vi "FindProjectElement.vi"(10 "Element name":string, 11 "Project item":refnum<vi>) -> (0 "Error":errorcluster, 2 "Found":bool, 3 "Element out":refnum<vi>)   [LabVIEW 2021, in "Tree.lvlib" / "Tree.lvclass"]
uses:
  Tree.lvclass
  Tree.lvclass/Tree.ctl
panel:
  # "Ищет в проекте объект (vi, класс, папка и т.д.) с названием Element name"
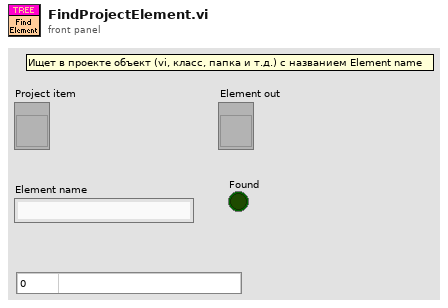
[diagram p1: front panel]
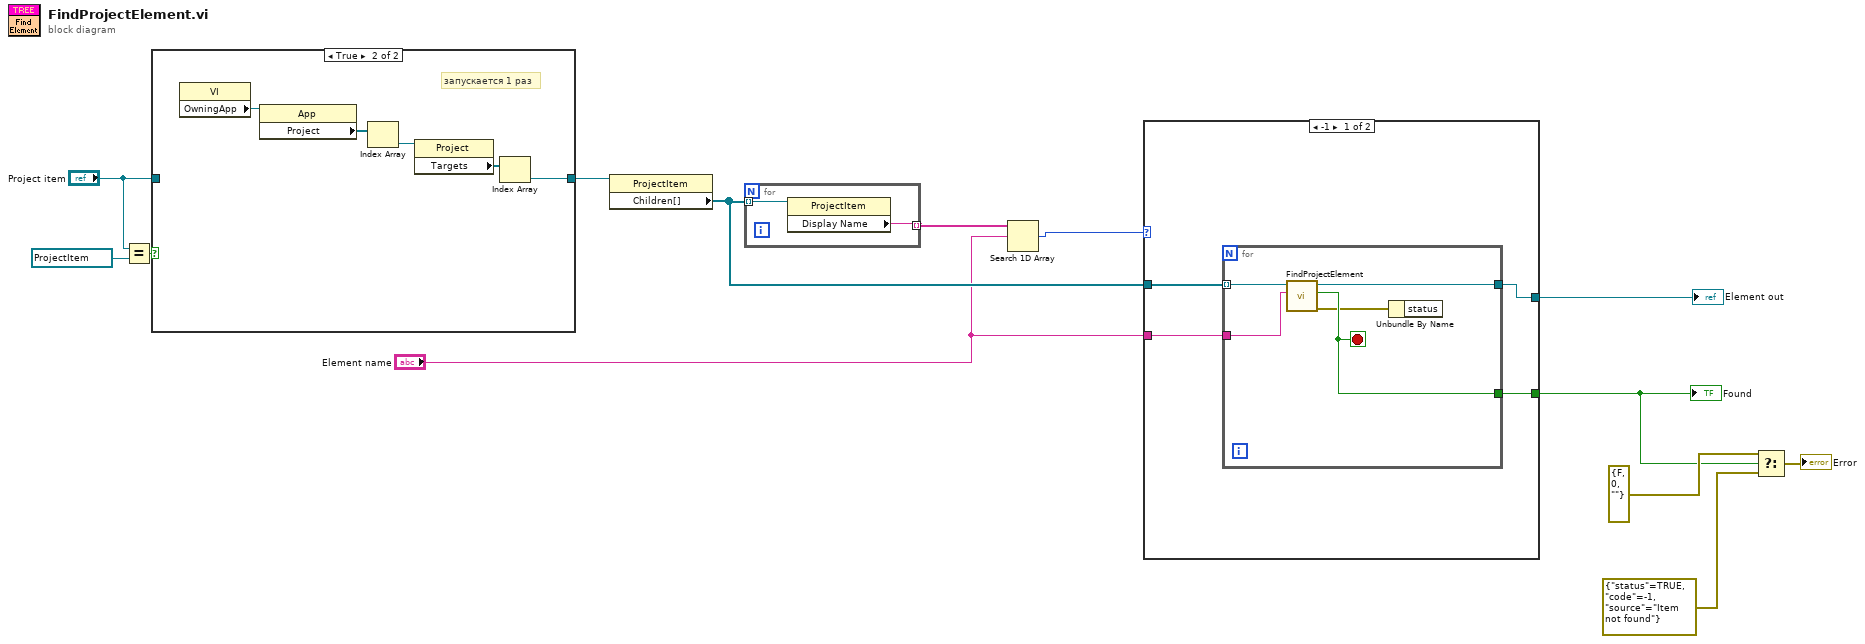
[diagram p0: block diagram]
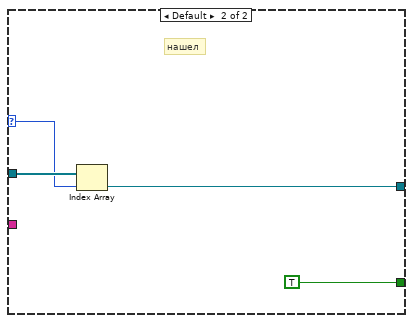
[diagram p3: hidden frame]
diagram:
  n1 = Equal?(x="Project item", y=refnum<vi> refnum) -> (x = y?=w3:bool)
  n2 = case shown="True" w3 {
    tunnel: [w14 w15] -> w2
    tunnel: "Project item" -> [w14 _]
    frame False {
    }
    frame True {
      # "запускается 1 раз"
      n3 = property class="VI"() -> ("OwningApp"=w16:refnum<vi>)  [unwired: 2 in, 2 out]
      n4 = property class="App"(reference=w16) -> ("Project"=w17:refnum<vi>[])  [unwired: 1 in, 2 out]
      n5 = Index Array(array=w17) -> (element=w18:refnum<vi>)  [unwired: 1 in]
      n6 = property class="Project"(reference=w18) -> ("Targets"=w19:refnum<vi>[])  [unwired: 1 in, 2 out]
      n7 = Index Array(array=w19) -> (element=w15:refnum<vi>)  [unwired: 1 in]
    }
  }
  n8 = property class="ProjectItem"(reference=w2) -> ("Children[]"=w11:refnum<vi>[])  [unwired: 1 in, 2 out]
  n9 = for {
    tunnel: w11 -> [w20] mode=indexing
    tunnel: [w21] -> w13 mode=indexing
    n10 = property class="ProjectItem"(reference=w20) -> ("Display Name"=w21:string)  [unwired: 1 in, 2 out]
  }
  n11 = Search 1D Array(1D array=w13, element="Element name") -> (index of element=w9:i32)  [unwired: 1 in]
  n12 = case shown="-1" w9 {
    selector: w9 -> [_ w31]
    tunnel: [w23 w34] -> w12
    tunnel: w11 -> [w25 w33]
    tunnel: "Element name" -> [w24 _]
    tunnel: [w22 TRUE ("Found")] -> w5
    frame -1 {
      n13 = for {
        tunnel: w25 -> [w30] mode=indexing
        tunnel: w24 -> [w29]
        tunnel: [w28] -> w23
        tunnel: [w27] -> w22
        stop <- w27 stop-if-true
        n14 = call "FindProjectElement.vi"("Element name"=w29, "Project item"=w30) -> ("Error"=w26:errorcluster, "Found"=w27:bool, "Element out"=w28:refnum<vi>)  [unwired: 7 in]
        n15 = Unbundle By Name(w26) -> ()  [unwired: 1 out]
      }
    }
    frame Default {
      # "нашел"
      n16 = Index Array(array=w33, index=w31) -> (element=w34:refnum<vi>)
    }
  }
  "Element out" <- w12
  "Found" <- w5
  n17 = Select(t=errorcluster {"status"=FALSE, "code"=0, "source"=""} ("error in (no error)"), s=w5, f=errorcluster {"status"=TRUE, "code"=-1, "source"="Item not found"} ("error in (no error)")) -> (s? t:f=→"Error":errorcluster)
